vi "MonitorServerMain.vi"() -> ()   [LabVIEW 2010, in "MonitorServer.lvlib"]
uses:
  MonitorServer.lvlib
  ModbusAddressRegister.ctl
  AutoChannelData.ctl
  DeviceListChannelData.ctl
  <vilib>/Utility/error.llb/DialogType.ctl
  Serial Config.ctl
  <vilib>/Utility/miscctls.llb/LVRectTypeDef.ctl
  DeviceListModbusAddressRegister.ctl
  SubVIs/ModBUS Driver/Private/MBDRV_Command List.ctl
  SubVIs/ModBUS Driver/Private/MBDRV_Command Data.ctl
  SubVIs/ModBUS Driver/Private/MBDRV_Action.ctl
  SubVIs/ModBUS Driver/Private/MBDRV_Response List.ctl
  SubVIs/ModBUS Driver/Private/MBDRV_Response.ctl
panel:
  out "error out":errorcluster
  out "source out":string
  out "message":string=" INSTRUCTIONS:\r\rNormal Use:  When using subVIs that incorporate the error in/error out (or error I/O) structure, place this handler where you want to inform the user of an error, typically at the end of the I/O data path, as the last action of the program.  If the error in error? is ERROR, the handler creates a message describing the error and its source.  If the type of dialog = 1 (default), the message is displayed to the user, who can only acknowedge it.  If the type = 2, the user can acknowledge the message or abort execution; aborting a program with active I/O is not recommended.  If the type = 0, no message is displayed; this is used to process the error programmatically, and the error out cluster elements are wired to individual terminals for that reason.  \r\rOther Use:\n\r\nlocal testing.  To test the error code of a subVI or function that does not have the error I/O structure, you can wire its error code and a source string to the local error code and error source inputs.  If error in error? indicates no error and error code is not equal to 0, the local code and source are substituted for the error in values, and error? is set TRUE (ERROR)."
  out "AutoReadChannels":T1
  in  "ChannelData":T2
  in  "Address":T3
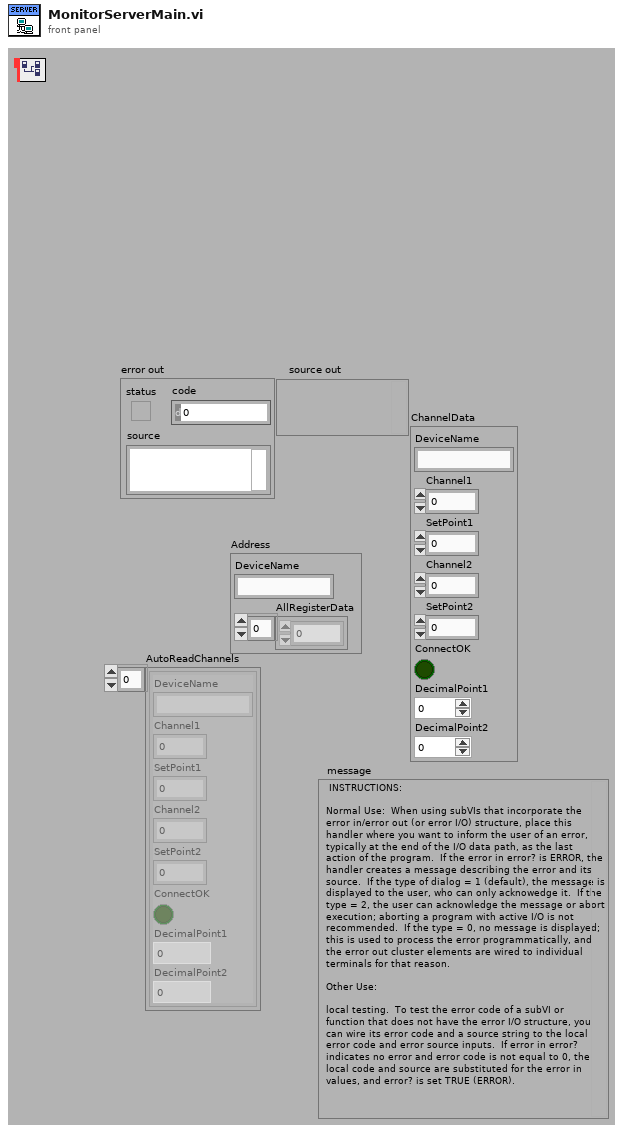
[diagram p1: front panel]
types:
  T1 = typedef "MonitorServer.lvlib/DeviceListChannelData.ctl" = T2[]
  T2 = typedef "MonitorServer.lvlib/AutoChannelData.ctl" = cluster{"DeviceName":string, "Channel1":dbl, "SetPoint1":dbl, "Channel2":dbl, "SetPoint2":dbl, "ConnectOK":bool, "DecimalPoint1":i16, "DecimalPoint2":i16}
  T3 = typedef "MonitorServer.lvlib/ModbusAddressRegister.ctl" = cluster{"DeviceName":string, "AllRegisterData":i16[]}
  T4 = enum32{"invalid app kind", "Development System", "Run Time System", "Student Edition", "Embedded LabVIEW", "Evaluation", "Custom"}
  T5 = typedef "LVRectTypeDef.ctl" = cluster{"Left":i16, "Top":i16, "Right":i16, "Bottom":i16}
  T6 = enum32{"Invalid", "Standard", "Closed", "Hidden", "Minimized", "Maximized"}
  T7 = typedef "MonitorServer.lvlib/Serial Config.ctl" = cluster{"设备名称":string, "串口选择":refnum<visa-resource-name>, "仪器地址":u32, "通讯速率":u32, "超时时间":u32, "刷新时间":dbl}
  T8 = cluster{"Core":cluster{"Current VI Reference":refnum<vi>, "Close Panel on Exit?":bool}, "Devices":T7[]}
  T9 = typedef "DialogType.ctl" = u16
  T10 = cluster{"Current VI Reference":refnum<vi>, "Close Panel on Exit?":bool}
  T11 = typedef "Path InitPaths__FS.ctl" = cluster{"Ctrller CFG":path, "INI":path, "Profile":path, "EventLog":path, "Data":path}
  T12 = typedef "MBDRV_Command List.ctl" = T13[]
  T13 = typedef "MBDRV_Command Data.ctl" = cluster{"Action":T14, "Com Port":string, "Register Address":u16, "Data To Write/Num To Read":i16}
  T14 = typedef "MBDRV_Action.ctl" = enum16{"Write", "Read"}
  T15 = typedef "MBDRV_Response List.ctl" = T16[]
  T16 = typedef "MBDRV_Response.ctl" = cluster{"Action":T14, "Com Port":string, "Register Address":u16, "Data":i16[]}
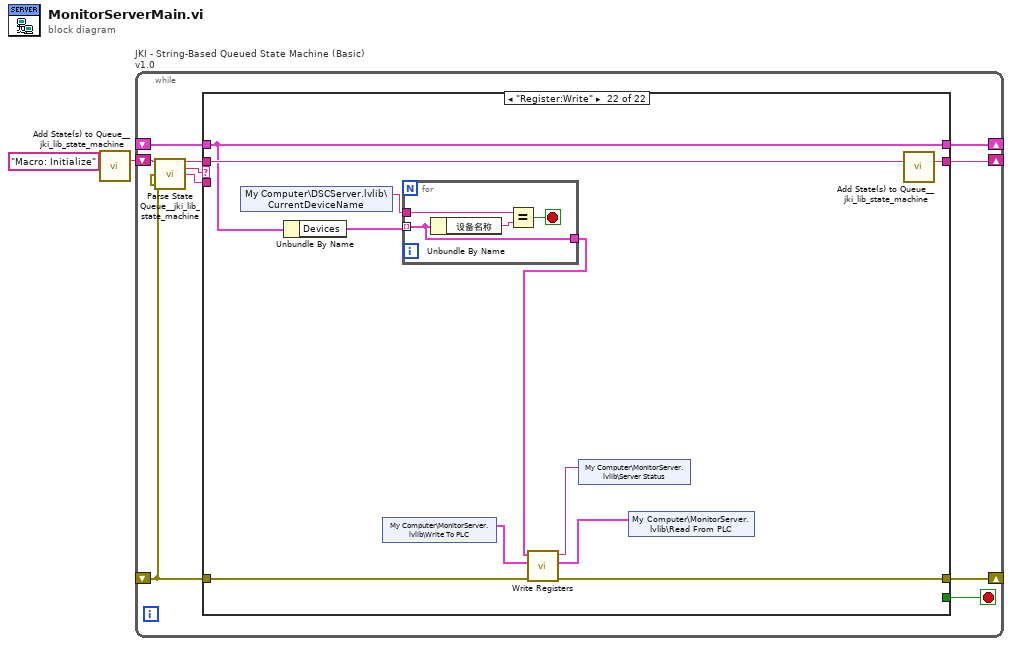
[diagram p0: block diagram]
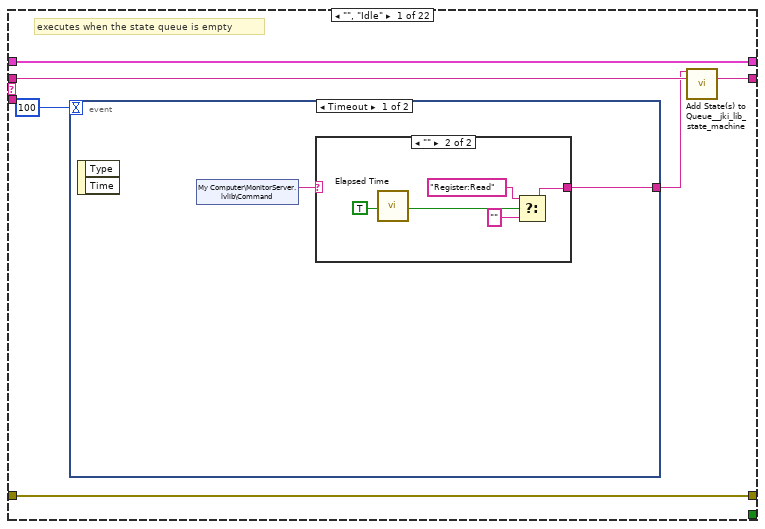
[diagram p2: hidden frame]
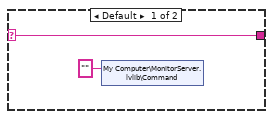
[diagram p3: hidden frame]
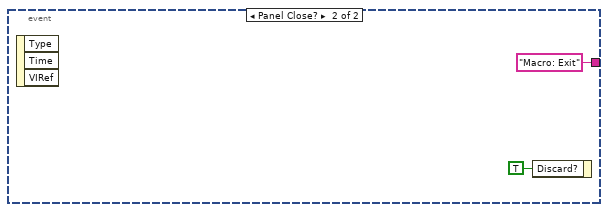
[diagram p4: hidden frame]
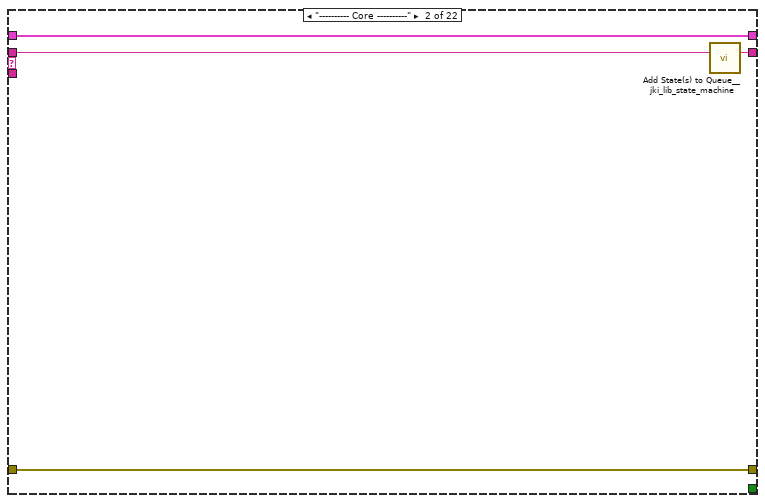
[diagram p5: hidden frame]
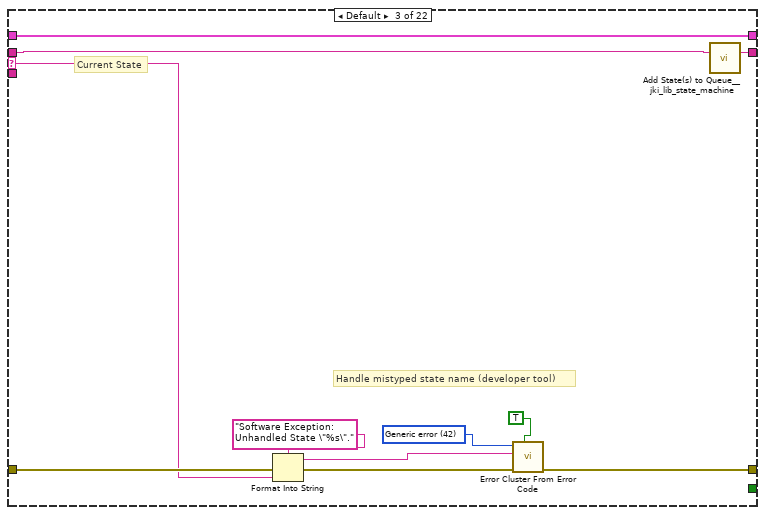
[diagram p6: hidden frame]
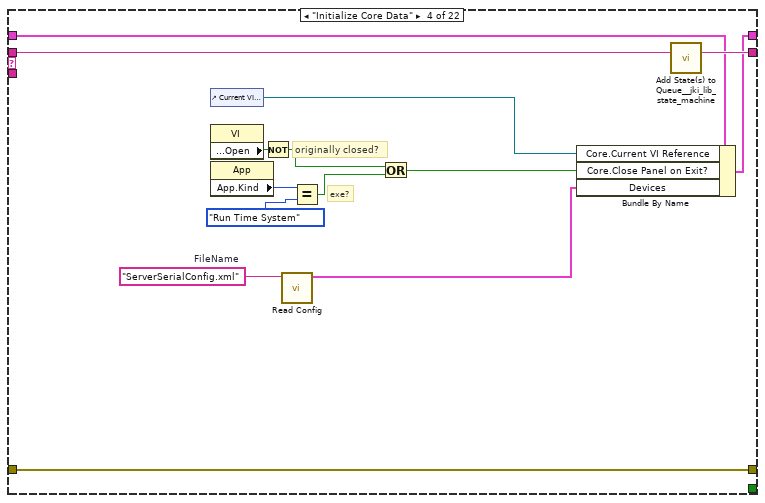
[diagram p7: hidden frame]
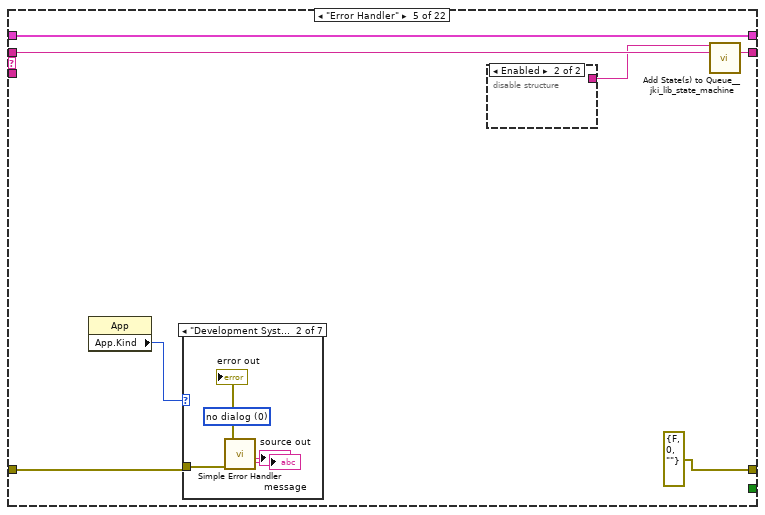
[diagram p8: hidden frame]
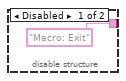
[diagram p15: hidden frame]
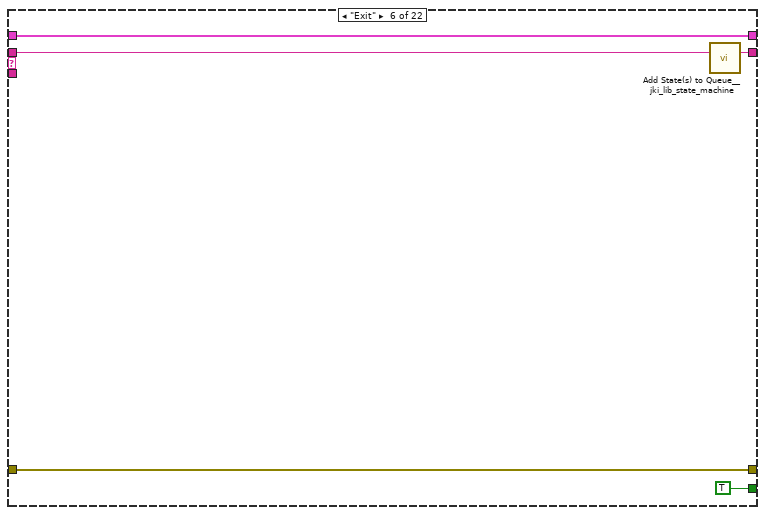
[diagram p16: hidden frame]
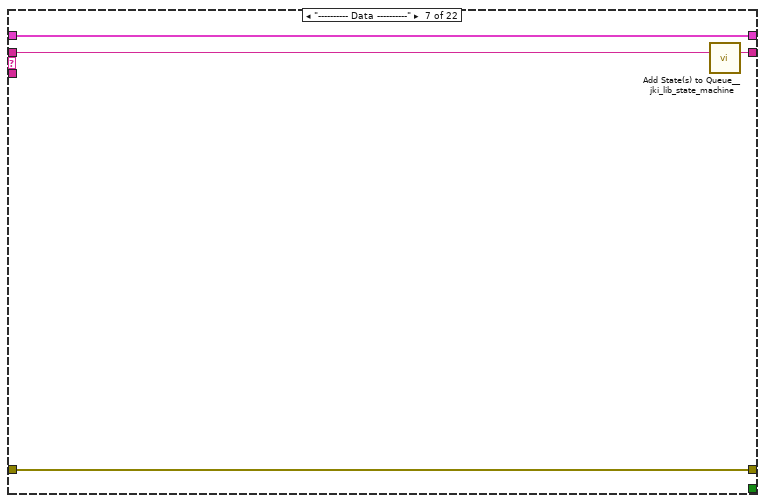
[diagram p17: hidden frame]
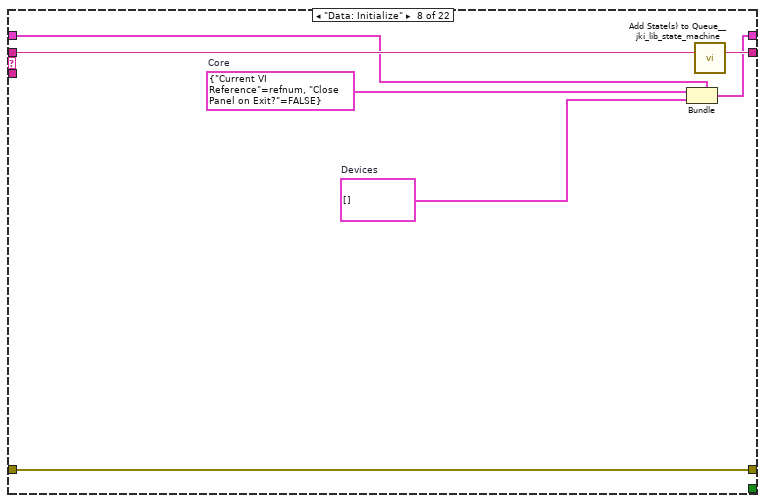
[diagram p18: hidden frame]
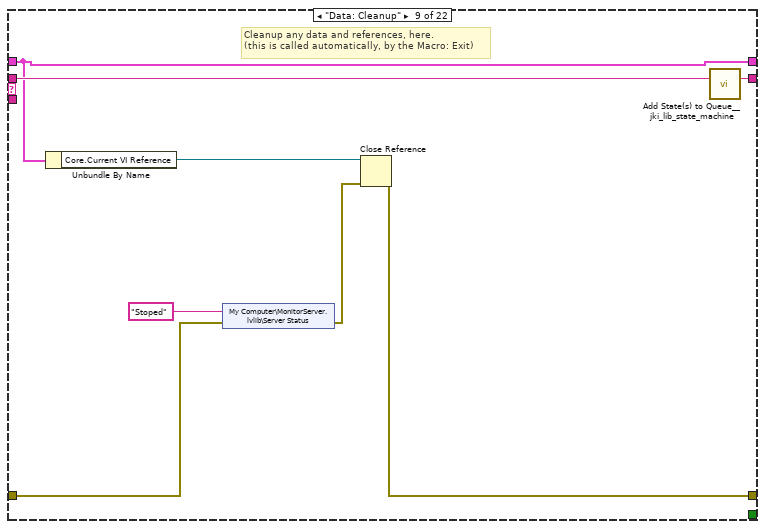
[diagram p19: hidden frame]
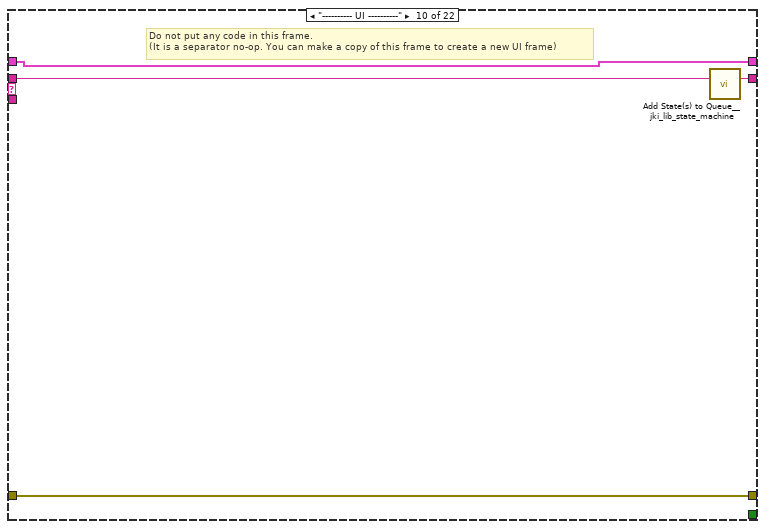
[diagram p20: hidden frame]
diagram:
  n1 = call "Add State(s) to Queue__jki_lib_state_machine.vi"("State(s) in (\"\")"="Macro: Initialize") -> ("States Out"=w2:string)  [unwired: 14 in]
  n2 = while "JKI - String-Based Queued State Machine (Basic) v1.0" {
    shift-right: [w5] -> _
    shift-left: _ -> [w4]
    shift-right: [w8] -> _
    shift-left: _ -> [w3]
    shift-right: [w7] -> _
    shift-left: w2 -> [w9]
    stop <- w6 stop-if-true
    n3 = call "Parse State Queue__jki_lib_state_machine.vi"("State Queue"=w9, "Error In (no error)"=w3) -> ("Remaining States"=w11:string, "Current State"=w12:string, "Arguments"=w10:string)  [unwired: 11 in]
    n4 = case shown="\"Register:Write\"" w12 {
      selector: w12 -> [_ _ w34 _ _ _ _ _ _ _ _ _ _ _ _ _ _ _ _ _ _ _]
      tunnel: w11 -> [w17 w33 w38 w58 w65 w75 w79 w86 w94 w98 w104 w112 w125 w155 w160 w170 w174 w179 w199 w212 w236 w254]
      tunnel: w10 -> [_ _ _ _ _ _ _ _ _ _ _ w107 w120 _ _ _ _ _ _ _ _ _]
      tunnel: w4 -> [w18 w30 w36 w48 w62 w73 w76 w81 w87 w95 w100 w110 w118 w152 w157 w161 w171 w176 w180 w207 w232 w244]
      tunnel: [w14 w31 w40 w56 errorcluster {"status"=FALSE, "code"=0, "source"=""} ("error out") w72 w77 w83 w91 w96 w102 w108 w122 w153 w158 w168 w172 w177 w185 w209 w228 w252] -> w8
      tunnel: w3 -> [w14 w31 w39 w56 w61 w72 w77 w83 w88 w96 w102 w109 w123 w153 w158 w168 w172 w177 w186 w210 w234 w248]
      tunnel: [w16 w32 w37 w57 w64 w74 w78 w85 w93 w97 w103 w111 w124 w154 w159 w169 w173 w178 w198 w211 w235 w253] -> w7
      tunnel: [_ _ _ _ _ TRUE _ _ _ _ _ _ _ _ _ _ _ _ _ _ _ _] -> w6
      tunnel: [w18 w30 w36 w47 w62 w73 w76 w82 w87 w95 w100 w110 w117 w152 w157 w161 w171 w176 w180 w207 w232 w244] -> w5
      frame "", "Idle" {
        # "executes when the state queue is empty"
        n5 = event shown="[0] Timeout" {
          selector: _ -> [_ _]
          dyn-events: _ -> [_ _]
          timeout: 100 -> [_ _]
          tunnel: [w19 "Macro: Exit" ("f")] -> w15
          event Timeout {
            n6 = event-data() -> ()  [unwired: 1 in, 2 out]
            n7 = shared-variable "My Computer\\MonitorServer.lvlib\\Command"() -> (w20:string)  [unwired: 1 in, 1 out]
            n8 = case shown="\"\"" w20 {
              selector: w20 -> [w22 _]
              tunnel: [w22 w27] -> w19
              frame Default {
                n9 = shared-variable "My Computer\\MonitorServer.lvlib\\Command"("" ("Command")) -> ()  [unwired: 1 in, 1 out]
              }
              frame "" {
                n10 = call "Elapsed Time"("Auto Reset"=TRUE) -> ("Time has Elapsed"=w25:bool)  [unwired: 11 in, 7 out]
                n11 = Select(t="Register:Read", s=w25, f="") -> (s? t:f=w27:string)
              }
            }
          }
          event Panel Close? {
            n12 = event-data() -> ()  [unwired: 1 in, 3 out]
            n13 = event-data("Discard?"=TRUE) -> ()  [unwired: 1 in, 1 out]
          }
        }
        n14 = call "Add State(s) to Queue__jki_lib_state_machine.vi"("State(s) in Front (\"\")"=w15, "State(s) in (\"\")"=w17) -> ("States Out"=w16:string)  [unwired: 13 in]
      }
      frame "---------- Core ----------" {
        n15 = call "Add State(s) to Queue__jki_lib_state_machine.vi"("State(s) in (\"\")"=w33) -> ("States Out"=w32:string)  [unwired: 14 in]
      }
      frame Default {
        w43 = 42 items=["No error", "Argument error", "Memory is full", "Out of zone", "End of file", "File already open", "Generic file I/O error", "File not found", "File permission error", "Disk is full", "Duplicate path", "Too many files open", "System feature not enabled", "Resource file not found", "Cannot add resource", "Resource not found", "Image not found", "Image memory error", "Pen does not exist", "Config type invalid", "Config token not found", "Config parse error", "Config memory error", "Bad external code format", "Bad external code offset", "External code not present", "Null window", "Destroy window error", "Null menu", "Print aborted", "Bad print record", "Print driver error", "Windows error during printing", "Memory error during printing", "Print dialog error", "Generic print error", "Invalid device refnum", "Device not found", "Device parameter error", "Device unit error", "Cannot open device", "Device call aborted", "Generic error", "Cancelled by user", "Object ID too low", "Object ID too high", "Object not in heap", "Unknown heap", "Unknown object (invalid DefProc)", "Unknown object (DefProc not in table)", "Message out of range", "Invalid (null) method", "Unknown message", "Manager call not supported", "Bad address", "Network operation in progress", "Network operation timed out", "Connection is busy", "Network attribute not supported", "Network error", "Address in use", "System out of memory", "Connection aborted", "Connection refused", "Not connected", "Already connected", "Connection closed", "Initialization error (interapplication manager)", "Bad occurrence", "Wait on unbound occurrence handler", "Occurrence queue overflow", "Datalog type conflict", "Unused", "Unrecognized type (interapplication manager)", "Memory corrupt", "Failed to make temporary DLL", "Old CIN version", "Drag socket not found", "Failed to load drop-object", "Failed to register OLE object", "Failed to release OLE object", "Format specifier type mismatch", "Unknown format specifier", "Too few format specifiers", "Too many format specifiers", "Scan failed", "Newer CIN version", "Error converting to variant", "Runtime menu error", "Password tampered", "Variant attribute not found", "Incompatible variant data type", "Event data is not available", "Event Store is not present", "Occurrence is not found", "Event Queue is not created", "Event info is not available", "Refnum passed is NULL", "Error retrieving Class GUID", "Error retrieving CoClass GUID", "Error retrieving TypeLib GUID.", "Bad built application magic bytes.", "Specific driver is different from the specific driver associated with the Logical Name.", "There is no session opened to the class driver.", "Max Error", "MAX - Error with config objects", "MAX - Error loading configuration", "MAX - Group not supported"]
        # "Current State"
        # "Handle mistyped state name (developer tool)"
        n16 = Format Into String(format string="Software Exception: Unhandled State \"%s\"." ("message"), error in=w39, w34) -> (resulting string=w42:string, error out=w41:errorcluster)  [unwired: 1 in]
        n17 = call <vilib>:"Error Cluster From Error Code.vi"("show call chain? (False)"=TRUE, "error in (no error)"=w41, "error message (\"\")"=w42, "error code (0)"=w43) -> ("error out"=w40:errorcluster)  [unwired: 5 in]
        n18 = call "Add State(s) to Queue__jki_lib_state_machine.vi"("State(s) in (\"\")"=w38) -> ("States Out"=w37:string)  [unwired: 14 in]
      }
      frame "Initialize Core Data" {
        w49 = "ServerSerialConfig.xml"  # FileName
        # "originally closed?"
        # "exe?"
        n19 = control-ref of="Current VI Reference"() -> (w45:refnum<vi>)
        n20 = property class="VI"() -> ("Front Panel.Open"=w55:bool)  [unwired: 2 in, 2 out]
        n21 = property class="App"() -> ("App.Kind"=w54:T4)  [unwired: 2 in, 2 out]
        n22 = Not(x=w55) -> (.not. x?=w52:bool)
        n23 = call "Read Config.vi"("ConfigurationFileName"=w49) -> ("DeviceList"=w46:T7[])  [unwired: 9 in, 1 out]
        n24 = Equal?(x=w54, y=T4."Run Time System" ("Application:Kind")) -> (x = y?=w51:bool)
        n25 = Or(x=w52, y=w51) -> (x .or. y?=w50:bool)
        n26 = Bundle By Name(cluster=w48, "Core.Current VI Reference"=w45, "Core.Close Panel on Exit?"=w50, "Devices"=w46) -> (w47:T8)
        n27 = call "Add State(s) to Queue__jki_lib_state_machine.vi"("State(s) in (\"\")"=w58) -> ("States Out"=w57:string)  [unwired: 14 in]
      }
      frame "Error Handler" {
        n28 = property class="App"() -> ("App.Kind"=w59:T4)  [unwired: 2 in, 2 out]
        n29 = case shown="\"Development System\", Default" w59 {
          tunnel: w61 -> [_ w69 _ _ _ _ _]
          frame "invalid app kind" {
          }
          frame "Development System", Default {
            w68 = T9 0 items=["no dialog", "OK message", "continue or stop message", "OK message + warnings", "continue/stop + warnings"] ("type of dialog (OK msg:1)")
            n30 = call <vilib>:"Simple Error Handler.vi"("type of dialog (OK msg:1)"=w68, "error in (no error)"=w69) -> ("source out"=→"source out":string, "message"=→"message":string)  [unwired: 3 in, 3 out]
            "error out" <- w69
          }
          frame "Run Time System" {
          }
          frame "Student Edition" {
          }
          frame "Embedded LabVIEW" {
          }
          frame "Evaluation" {
          }
          frame "Custom" {
          }
        }
        n31 = disable-structure shown="Enabled" {
          disable-tunnel: ["Macro: Exit" _] -> w60
          frame Disabled {
          }
          frame Enabled {
          }
        }
        n32 = call "Add State(s) to Queue__jki_lib_state_machine.vi"("State(s) in Front (\"\")"=w60, "State(s) in (\"\")"=w65) -> ("States Out"=w64:string)  [unwired: 13 in]
      }
      frame "Exit" {
        n33 = call "Add State(s) to Queue__jki_lib_state_machine.vi"("State(s) in (\"\")"=w75) -> ("States Out"=w74:string)  [unwired: 14 in]
      }
      frame "---------- Data ----------" {
        n34 = call "Add State(s) to Queue__jki_lib_state_machine.vi"("State(s) in (\"\")"=w79) -> ("States Out"=w78:string)  [unwired: 14 in]
      }
      frame "Data: Initialize" {
        w80 = T7[] []  # Devices
        w84 = T10 {"Current VI Reference"=refnum, "Close Panel on Exit?"=FALSE}  # Core
        n35 = Bundle(cluster=w81, "Core"=w84, "Devices"=w80) -> (w82:T8)
        n36 = call "Add State(s) to Queue__jki_lib_state_machine.vi"("State(s) in (\"\")"=w86) -> ("States Out"=w85:string)  [unwired: 14 in]
      }
      frame "Data: Cleanup" {
        # "Cleanup any data and references, here.\n(this is called automatically, by the Macro: Exit)"
        n37 = Unbundle By Name(w87) -> ("Core.Current VI Reference"=w92:refnum<vi>)
        n38 = shared-variable "My Computer\\MonitorServer.lvlib\\Server Status"("Stoped" ("Server Status"), error in=w88) -> (error out=w89:errorcluster)
        n39 = Close Reference(reference=w92, error in (no error)=w89) -> (error out=w91:errorcluster)
        n40 = call "Add State(s) to Queue__jki_lib_state_machine.vi"("State(s) in (\"\")"=w94) -> ("States Out"=w93:string)  [unwired: 14 in]
      }
      frame "---------- UI ----------" {
        # "Do not put any code in this frame.\n(It is a separator no-op. You can make a copy of this frame to create a new UI frame)"
        n41 = call "Add State(s) to Queue__jki_lib_state_machine.vi"("State(s) in (\"\")"=w98) -> ("States Out"=w97:string)  [unwired: 14 in]
      }
      frame "UI: Initialize" {
        # "Initialize the User Interface, here.\n(this is called automatically, by the Macro: Init)"
        n42 = Unbundle By Name(w100) -> ("Core.Current VI Reference"=w101:refnum<vi>)
        n43 = property class="App"() -> ("App.Kind"=w99:T4)  [unwired: 2 in, 2 out]
        n44 = case shown="\"invalid app kind\", Default" w99 {
          tunnel: w101 -> [w105 _]
          frame "invalid app kind", Default {
            n45 = property class="VI"(reference=w105, "Front Panel.WinBounds"=T5 {"Left"=0, "Top"=0, "Right"=1, "Bottom"=1} ("Front Panel Window:Window Bounds")) -> ()  [unwired: 1 in, 2 out]
          }
          frame "Development System" {
          }
        }
        n46 = call "Add State(s) to Queue__jki_lib_state_machine.vi"("State(s) in (\"\")"=w104) -> ("States Out"=w103:string)  [unwired: 14 in]
      }
      frame "UI: Cursor Set" {
        # "Argument"
        # "Set and Unset Cursor Busy.\n(Usage: \"UI: Cursor Set >> Busy|Idle\")"
        n47 = case shown="\"Idle\", Default" w107 {
          tunnel: w109 -> [w114 w116]
          tunnel: [w113 w115] -> w108
          frame "Idle", Default {
            n48 = call <vilib>:"Unset Busy.vi"("error in (no error)"=w114) -> ("error out"=w113:errorcluster)  [unwired: 10 in]
          }
          frame "Busy" {
            n49 = call <vilib>:"Set Busy.vi"("error in (no error)"=w116) -> ("error out"=w115:errorcluster)  [unwired: 9 in, 1 out]
          }
        }
        n50 = call "Add State(s) to Queue__jki_lib_state_machine.vi"("State(s) in (\"\")"=w112) -> ("States Out"=w111:string)  [unwired: 14 in]
      }
      frame "UI: Front Panel State" {
        # "Argument"
        # "Set Front Panel Open or Closed\n(Usage: \"UI: Front Panel State >> Open|Close\")"
        n51 = Unbundle By Name(w118) -> ("Core.Current VI Reference"=w121:refnum<vi>)
        n52 = case shown="\"Open\", Default" w120 {
          tunnel: w123 -> [w130 w144]
          tunnel: [w131 w145] -> w122
          tunnel: w121 -> [_ _]
          tunnel: [w126 w140] -> w119
          frame "Open", Default {
            n53 = property class="VI"(error in=w130) -> (reference out=w128:refnum<vi>, error out=w129:errorcluster, "Front Panel.Open"=w127:bool)  [unwired: 1 in]
            n54 = case shown="True" w127 {
              tunnel: [w135 w139] -> w131
              tunnel: w129 -> [w134 w139]
              tunnel: w128 -> [w133 w138]
              tunnel: [w132 w138] -> w126
              frame False {
                n55 = invoke class="VI" method="FP.Open"(reference=w133, error in=w134, "Activate"=TRUE, "State"=T6."Standard") -> (reference out=w132:refnum<vi>, error out=w135:errorcluster)  [unwired: 1 in, 3 out]
              }
              frame True {
              }
            }
          }
          frame "Close" {
            n56 = property class="VI"(error in=w144) -> (reference out=w142:refnum<vi>, error out=w143:errorcluster, "Front Panel.Open"=w141:bool)  [unwired: 1 in]
            n57 = case shown="True" w141 {
              tunnel: [w147 w151] -> w145
              tunnel: w143 -> [w147 w150]
              tunnel: w142 -> [w146 w149]
              tunnel: [w146 w148] -> w140
              frame False {
              }
              frame True {
                n58 = invoke class="VI" method="FP.Close"(reference=w149, error in=w150) -> (reference out=w148:refnum<vi>, error out=w151:errorcluster)  [unwired: 1 in, 1 out]
              }
            }
          }
        }
        n59 = Bundle By Name(cluster=w118, "Core.Current VI Reference"=w119) -> (w117:T8)
        n60 = call "Add State(s) to Queue__jki_lib_state_machine.vi"("State(s) in (\"\")"=w125) -> ("States Out"=w124:string)  [unwired: 14 in]
      }
      frame "---------- Macro ----------" {
        # "Do not put any code in this frame.\n(It is a separator no-op. You can make a copy of this frame to create a new Macro frame)"
        n61 = call "Add State(s) to Queue__jki_lib_state_machine.vi"("State(s) in (\"\")"=w155) -> ("States Out"=w154:string)  [unwired: 14 in]
      }
      frame "Macro: Initialize" {
        w156 = "Data: Initialize\nInitialize Core Data\nUI: Initialize\nUI: Front Panel State >> Open\nRegister:ReadAll\nDelay"  # Data: Initialize Initialize Core Data UI: Initialize UI: Front Panel State >> Open Register:ReadAll Delay
        # "Initialization Macro\n(This is called once, when the VI starts)"
        n62 = call "Add State(s) to Queue__jki_lib_state_machine.vi"("State(s) in Front (\"\")"=w156, "State(s) in (\"\")"=w160) -> ("States Out"=w159:string)  [unwired: 13 in]
      }
      frame "Macro: Exit" {
        n63 = Unbundle By Name(w161) -> ("Core.Close Panel on Exit?"=w162:bool)
        n64 = Select(t="UI: Front Panel State >> Close", s=w162, f="") -> (s? t:f=w165:string)
        n65 = call "Add State(s) to Queue__jki_lib_state_machine.vi"("State(s) in (\"\")"=w165, "State(s) at Back (\"\")"="Data: Cleanup\nExit") -> ("States Out"=w163:string)  [unwired: 13 in]
        n66 = call "Add State(s) to Queue__jki_lib_state_machine.vi"("State(s) in Front (\"\")"=w163, "State(s) in (\"\")"=w170) -> ("States Out"=w169:string)  [unwired: 13 in]
      }
      frame "---------- New Category ----------" {
        # "Template Separator\n(You can make a copy of, or modify, this frame)"
        n67 = call "Add State(s) to Queue__jki_lib_state_machine.vi"("State(s) in (\"\")"=w174) -> ("States Out"=w173:string)  [unwired: 14 in]
      }
      frame "Delay" {
        # "Template Separator\n(You can make a copy of, or modify, this frame)"
        n68 = Wait (ms)(milliseconds to wait=u32 100) -> ()  [unwired: 1 out]
        n69 = call "Add State(s) to Queue__jki_lib_state_machine.vi"("State(s) in (\"\")"=w179) -> ("States Out"=w178:string)  [unwired: 14 in]
      }
      frame "Profile:Download" {
        n70 = shared-variable "My Computer\\DSCServer.lvlib\\CurrentDeviceName"() -> (w183:string)  [unwired: 1 in, 1 out]
        n71 = call "File System Paths__FS.vi"("error in (no error)"=w186) -> ("error out"=w187:errorcluster, "FilePaths"=w194:T11)  [unwired: 8 in, 1 out]
        n72 = Unbundle By Name(w194) -> ("Profile"=w196:path)
        n73 = Unbundle By Name(w180) -> ("Devices"=w184:T7[])
        n74 = Build Path(base path=w196, name or relative path="Default.pfl" ("默认名称")) -> (appended path=w195:path)
        n75 = call "Profile Read__FS.vi"("error in (no error)"=w187, "路径"=w195) -> ("error out"=w188:errorcluster, "Item Names"=w191:string[][])  [unwired: 7 in, 1 out]
        n76 = for {
          tunnel: w184 -> [w205] mode=indexing
          tunnel: w183 -> [w203]
          tunnel: [w201] -> w182
          tunnel: [w200] -> w181
          stop <- w202 stop-if-true
          n77 = Unbundle By Name(w205) -> ("设备名称"=w204:string, "串口选择"=w201:refnum<visa-resource-name>, "仪器地址"=w200:u32)
          n78 = Equal?(x=w203, y=w204) -> (x = y?=w202:bool)
        }
        n79 = call "Global Variable Item Names__PD.vi"("Inqueue?"=TRUE, "error in (no error)"=w188, "Mesages"=w191) -> ("error out"=w192:errorcluster)  [unwired: 7 in, 1 out]
        n80 = call "Global Variable Item Names__PD.vi"("error in (no error)"=w192) -> ("error out"=w189:errorcluster, "Message Out"=w190:string[][])  [unwired: 9 in]
        n81 = call "Profile Communication__PD.vi"("Unit Address (1)"=w181, "error in (no error)"=w189, "Events"=w190, "VISA resource name out"=w182) -> ("error out"=w185:errorcluster)  [unwired: 7 in]
        n82 = call "Add State(s) to Queue__jki_lib_state_machine.vi"("State(s) in (\"\")"=w199) -> ("States Out"=w198:string)  [unwired: 14 in]
      }
      frame "Register:Read" {
        n83 = Unbundle By Name(w207) -> ("Devices"=w208:T7[])
        n84 = for {
          tunnel: w210 -> [w227]
          tunnel: [w217] -> w209
          tunnel: w208 -> [w225] mode=indexing
          tunnel: [w218] -> w206 mode=indexing
          n85 = Unbundle By Name(w225) -> ("设备名称"=w224:string)
          n86 = call "Read Registers.vi"("error in (no error)"=w227, "Serial Config"=w225) -> ("error out"=w226:errorcluster, "DecimalPoint2"=w213:i16, "DecimalPoint1"=w214:i16, "SP 2"=w220:dbl, "Input2 Value"=w221:dbl, "SP 1"=w222:dbl, "Input1 Value"=w223:dbl)  [unwired: 2 in, 1 out]
          n87 = call "DataLog.vi"("CH2 SP"=w220, "CH1 SP"=w222, "error in (no error)"=w226, "CH2"=w221, "CH1"=w223, "Controller Name"=w224) -> ("error out"=w217:errorcluster)  [unwired: 5 in]
          n88 = Unbundle By Name(w217) -> ("status"=w216:bool)
          n89 = Not(x=w216) -> (.not. x?=w215:bool)
          n90 = Bundle(cluster="ChannelData", "DeviceName"=w224, "Channel1"=w223, "SetPoint1"=w222, "Channel2"=w221, "SetPoint2"=w220, "ConnectOK"=w215, "DecimalPoint1"=w214, "DecimalPoint2"=w213) -> (w218:T2)
        }
        "AutoReadChannels" <- w206
        n91 = shared-variable "My Computer\\MonitorServer.lvlib\\AutoReadChannels"(w206) -> ()  [unwired: 1 in, 1 out]
        n92 = call "Add State(s) to Queue__jki_lib_state_machine.vi"("State(s) in (\"\")"=w212) -> ("States Out"=w211:string)  [unwired: 14 in]
      }
      frame "Register:ReadAll" {
        n93 = Unbundle By Name(w232) -> ("Devices"=w233:T7[])
        n94 = for {
          tunnel: w234 -> [w242]
          tunnel: [w241] -> w230 mode=indexing
          tunnel: w233 -> [w243] mode=indexing
          tunnel: [w237] -> w231 mode=indexing
          n95 = Unbundle By Name(w243) -> ("设备名称"=w240:string)
          n96 = call "ReadAllRegisters.vi"("error in (no error)"=w242, "Serial Config"=w243) -> ("error out"=w241:errorcluster, "AllRegisterData"=w239:i16[])  [unwired: 8 in]
          n97 = Bundle(cluster="Address", "DeviceName"=w240, "AllRegisterData"=w239) -> (w237:T3)
        }
        n98 = Merge Errors(w230) -> (w229:errorcluster)
        n99 = shared-variable "My Computer\\MonitorServer.lvlib\\DeviceListRegister"(w231, error in=w229) -> (error out=w228:errorcluster)
        n100 = call "Add State(s) to Queue__jki_lib_state_machine.vi"("State(s) in (\"\")"=w236) -> ("States Out"=w235:string)  [unwired: 14 in]
      }
      frame "Register:Write" {
        n101 = shared-variable "My Computer\\DSCServer.lvlib\\CurrentDeviceName"() -> (w246:string)  [unwired: 1 in, 1 out]
        n102 = Unbundle By Name(w244) -> ("Devices"=w247:T7[])
        n103 = shared-variable "My Computer\\MonitorServer.lvlib\\Write To PLC"() -> (w250:T12)  [unwired: 1 in, 1 out]
        n104 = for {
          tunnel: w247 -> [w255] mode=indexing
          tunnel: w246 -> [w257]
          tunnel: [w255] -> w245
          stop <- w256 stop-if-true
          n105 = Unbundle By Name(w255) -> ("设备名称"=w258:string)
          n106 = Equal?(x=w257, y=w258) -> (x = y?=w256:bool)
        }
        n107 = call "Write Registers.vi"("error in (no error)"=w248, "Command List"=w250, "Serial Config"=w245) -> ("error out"=w252:errorcluster, "Response List"=w251:T15, "Status Code"=w249:string)  [unwired: 6 in]
        n108 = shared-variable "My Computer\\MonitorServer.lvlib\\Server Status"(w249) -> ()  [unwired: 1 in, 1 out]
        n109 = shared-variable "My Computer\\MonitorServer.lvlib\\Read From PLC"(w251) -> ()  [unwired: 1 in, 1 out]
        n110 = call "Add State(s) to Queue__jki_lib_state_machine.vi"("State(s) in (\"\")"=w254) -> ("States Out"=w253:string)  [unwired: 14 in]
      }
    }
  }
